vi "Spectral Integration Fast Version.vi"() -> ()   [LabVIEW 2018]
uses:
  <vilib>/Utility/file.llb/Write To Spreadsheet File (string).vi
  <vilib>/Utility/file.llb/Write To Spreadsheet File (DBL).vi
  <instrlib>/Ocean Optics 2000 4000/Ocean Optics 2000 4000.lvlib
panel:
  in  "?":bool
  out "Calculated Dlambda":dbl[][](array[numeric])
  in  "Number of Measurements":dbl=50.0
  out "Spectrum Data":dbl[][](array[numeric])
  in  "File Name":string="Example.xls" caption="add .xls for excel or .tdms, etc"
  in  "Enable Spectrum Log":bool caption="Log Data"
  out "x dlambda":dbl[](array[numeric])
  out "Spectrum":dbl[](array[numeric])
  in  "dlambda, pm, default 271pm":dbl=271.0
  out "Spectrum by Pixel Number":dbl[](array[numeric])
  out "Wavelength (nm)":dbl[](array[numeric])
  out "Spectral Integration":dbl
  in  "Integration Time, ms":dbl=100.0
  in  "Enable Strobe (Disabled)":bool
  out "Spectral Waveform":cluster{dbl[], dbl[]}(graph)
  in  "VISA resource name":refnum<visa-resource-name>
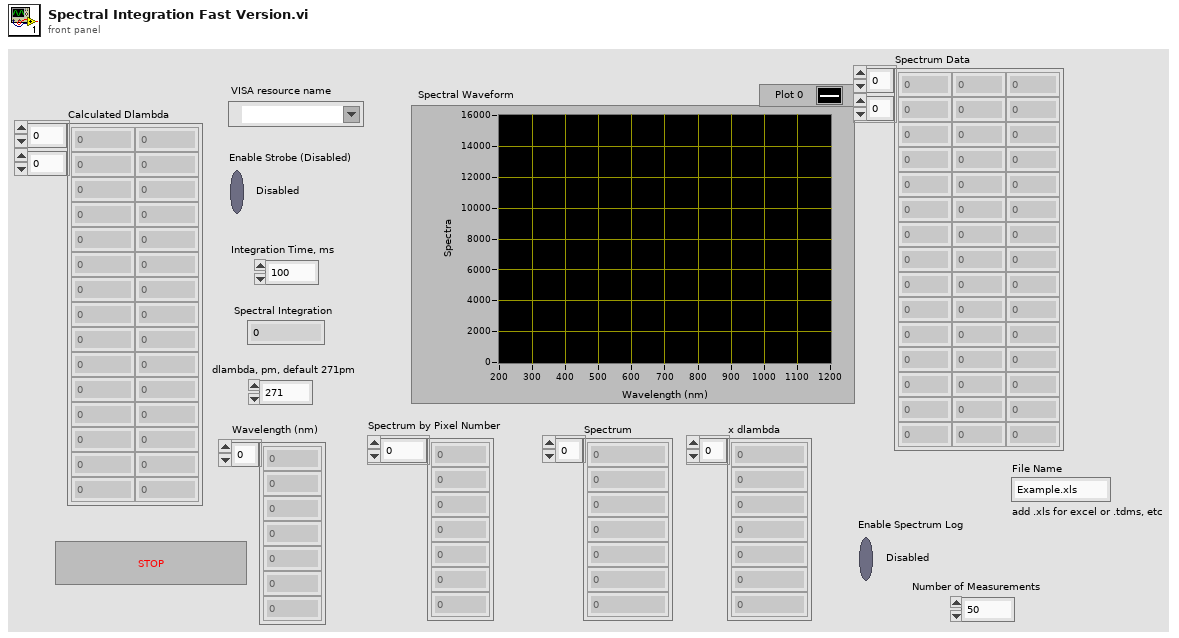
[diagram p1: front panel]
types:
  T1 = cluster{"Wavelength (nm)":dbl[], "Spectrum by Pixel Number":dbl[]}
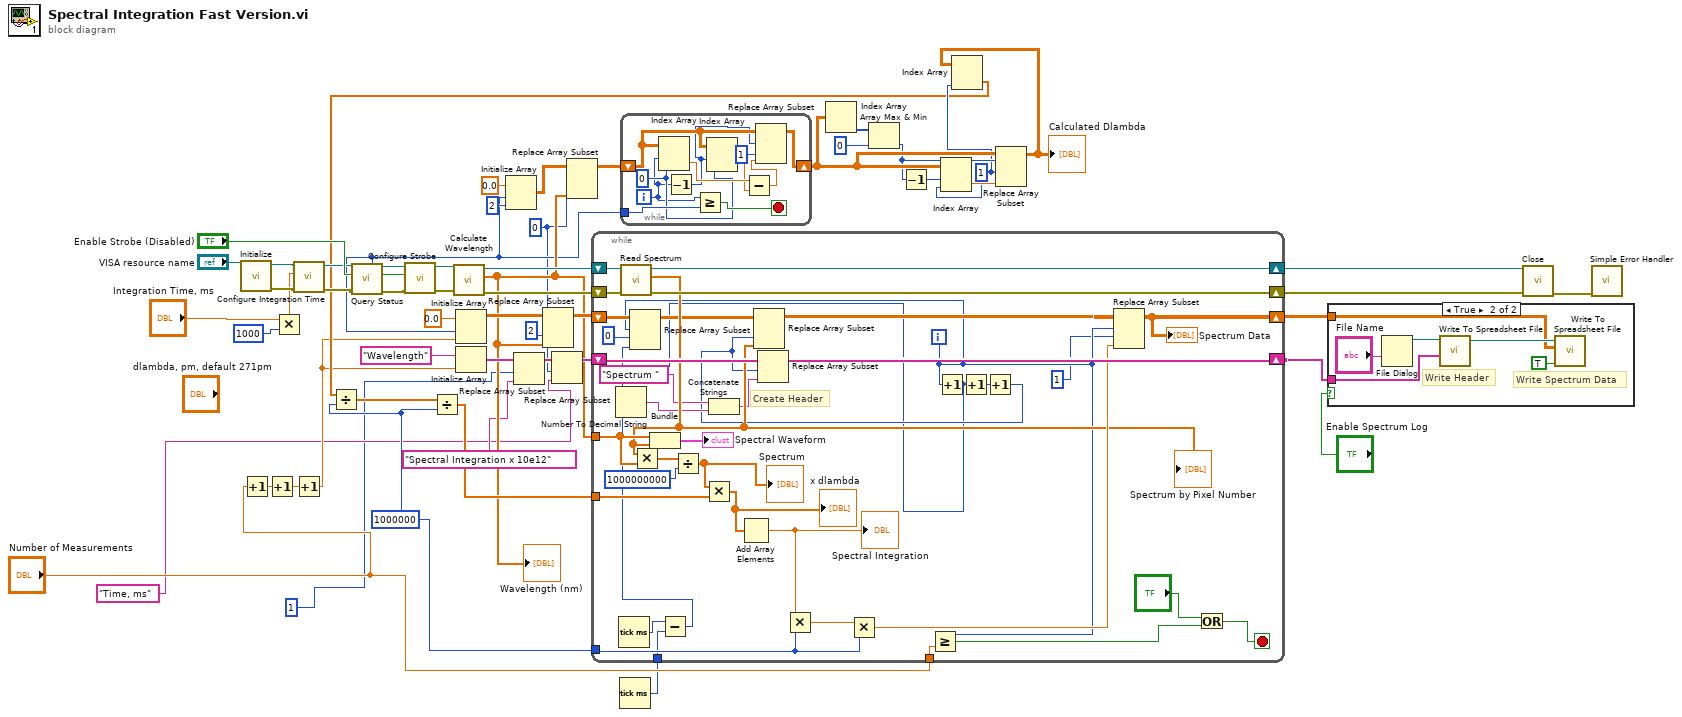
[diagram p0: block diagram]
diagram:
  w16 = 1
  w3 = 0
  w28 = 1000000
  n1 = call <instrlib>:"Initialize.vi"("VISA resource name"="VISA resource name") -> ("error out"=w51:errorcluster, "VISA resource name out"=w52:refnum<visa-resource-name>)  [unwired: 2 in, 7 out]
  n2 = Increment(x="Number of Measurements") -> (x+1=w1:dbl)
  n3 = Increment(x=w1) -> (x+1=w10:dbl)
  n4 = Multiply(x="Integration Time, ms", y=1000) -> (x*y=w48:dbl)
  n5 = call <instrlib>:"Configure Integration Time.vi"("error in (no error)"=w51, "Integration Time (6000)"=w48, "VISA resource name"=w52) -> ("error out"=w46:errorcluster, "VISA resource name out"=w44:refnum<visa-resource-name>)  [unwired: 7 in]
  n6 = Increment(x=w10) -> (x+1=w11:dbl)
  n7 = call <instrlib>:"Query Status.vi"("VISA resource name"=w44, "error in (no error)"=w46) -> ("Number of Pixels"=w14:u16, "VISA resource name out"=w43:refnum<visa-resource-name>, "error out"=w45:errorcluster)  [unwired: 11 out]
  n8 = call <instrlib>:"Configure Strobe.vi"("error in (no error)"=w45, "Enable Strobe (Disabled)"="Enable Strobe (Disabled)", "VISA resource name"=w43) -> ("error out"=w53:errorcluster, "VISA resource name out"=w54:refnum<visa-resource-name>)  [unwired: 7 out]
  n9 = call <instrlib>:"Calculate Wavelength.vi"("error in (no error)"=w53, "VISA resource name"=w54) -> ("error out"=w41:errorcluster, "Wavelength (nm)"=w15:dbl[], "VISA resource name out"=w42:refnum<visa-resource-name>)  [unwired: 1 in, 6 out]
  "Wavelength (nm)" <- w15
  n10 = Initialize Array(0.0 ("element"), w14, w11) -> (w36:dbl[][])
  n11 = Initialize Array("Wavelength", w11) -> (w30:string[])
  n12 = Initialize Array(0.0 ("element"), w14, 2) -> (w25:dbl[][])
  n13 = Replace Array Subset(array=w36, new element=w15, index (col)=2) -> (w35:dbl[][])  [unwired: 1 in]
  n14 = Replace Array Subset(array=w25, new element=w15, index (col)=w3) -> (w24:dbl[][])  [unwired: 1 in]
  n15 = Tick Count (ms)() -> (millisecond timer value=w9:u32)
  n16 = while {
    tunnel: w14 -> [w67]
    shift-right: [w61] -> w20
    shift-left: w24 -> [w63]
    i -> [w57]
    stop <- w66 stop-if-true
    w62 = 0
    n17 = Index Array(array=w63, index (row)=w57, index (col)=w62) -> (element=w65:dbl)
    n18 = Decrement(x=w57) -> (x-1=w58:i32)
    n19 = Greater Or Equal?(x=w57, y=w67) -> (x >= y?=w66:bool)
    n20 = Index Array(array=w63, index (row)=w58, index (col)=w62) -> (element=w64:dbl)
    n21 = Subtract(x=w65, y=w64) -> (x-y=w59:dbl)
    n22 = Replace Array Subset(array=w63, new element=w59, index (row)=w58, index (col)=1) -> (w61:dbl[][])
  }
  n23 = Array Max & Min(array=w20) -> (min index (indices)=w23:i32[])  [unwired: 3 out]
  n24 = Index Array(array=w23, index=0) -> (element=w18:i32)
  n25 = Decrement(x=w18) -> (x-1=w22:i32)
  n26 = Index Array(array=w20, index (row)=w22, index (col)=w16) -> (element=w21:dbl)
  n27 = Replace Array Subset(array=w20, new element=w21, index (row)=w18, index (col)=w16) -> (w19:dbl[][])
  "Calculated Dlambda" <- w19
  n28 = Index Array(array=w19, index (col)=w16) -> (element=w13:dbl[])  [unwired: 1 in]
  n29 = Divide(x=w13, y=w28) -> (x/y=w37:dbl[])
  n30 = Divide(x=w37, y=w28) -> (x/y=w34:dbl[])
  n31 = while {
    tunnel: w15 -> [w98]
    tunnel: w34 -> [w103]
    tunnel: w28 -> [w94]
    shift-right: [w86] -> w40
    shift-left: w42 -> [w90]
    shift-right: [w88] -> w39
    shift-left: w41 -> [w91]
    shift-right: [w97] -> w29
    shift-left: w35 -> [w92]
    tunnel: "Number of Measurements" -> [w80]
    tunnel: w9 -> [w78]
    shift-right: [w73] -> w8
    shift-left: w30 -> [w93]
    i -> [w74]
    stop <- w68 stop-if-true
    # "Create Header"
    n32 = Tick Count (ms)() -> (millisecond timer value=w81:u32)
    n33 = call <instrlib>:"Read Spectrum.vi"("error in (no error)"=w91, "VISA resource name"=w90) -> ("error out"=w88:errorcluster, "Spectrum by Pixel Number"=w87:dbl[], "VISA resource name out"=w86:refnum<visa-resource-name>)  [unwired: 6 in, 1 out]
    "Spectrum by Pixel Number" <- w87
    n34 = Multiply(x=w87, y=w98) -> (x*y=w101:dbl[])
    n35 = Bundle("Wavelength (nm)"=w98, "Spectrum by Pixel Number"=w87) -> (→"Spectral Waveform":T1)  [unwired: 1 out]
    n36 = Subtract(x=w81, y=w78) -> (x-y=w76:u32)
    n37 = Replace Array Subset(array=w92, new element=w76, index (row)=w74, index (col)=0) -> (w77:dbl[][])
    n38 = Divide(x=w101, y=1000000000) -> (x/y=w99:dbl[])
    "Spectrum" <- w99
    n39 = Multiply(x=w99, y=w103) -> (x*y=w104:dbl[])
    "x dlambda" <- w104
    n40 = Add Array Elements(numeric array=w104) -> (sum=w102:dbl)
    "Spectral Integration" <- w102
    n41 = Multiply(x=w102, y=w94) -> (x*y=w96:dbl)
    n42 = Multiply(x=w96, y=w94) -> (x*y=w95:dbl)
    n43 = Greater Or Equal?(x=w74, y=w80) -> (x >= y?=w70:bool)
    n44 = Increment(x=w74) -> (x+1=w71:i32)
    n45 = Number To Decimal String(number=w71) -> (decimal integer string=w85:string)  [unwired: 1 out]
    n46 = Concatenate Strings("Spectrum " ("string"), w85) -> (w83:string)
    n47 = Increment(x=w71) -> (x+1=w79:i32)
    n48 = Increment(x=w79) -> (x+1=w82:i32)
    n49 = Replace Array Subset(array=w77, new element=w87, index (col)=w82) -> (w89:dbl[][])  [unwired: 1 in]
    n50 = Replace Array Subset(array=w93, new element=w83, index=w82) -> (w73:string[])
    n51 = Replace Array Subset(array=w89, new element=w95, index (row)=w74, index (col)=1) -> (w97:dbl[][])
    "Spectrum Data" <- w97
    n52 = Or(x="?", y=w70) -> (x .or. y?=w68:bool)
  }
  n53 = Replace Array Subset(array=w8, new element="Spectral Integration x 10e12" ("string"), index=1) -> (w7:string[])
  n54 = Replace Array Subset(array=w7, new element="Time, ms" ("string"), index=w3) -> (w5:string[])
  n55 = case shown="True" "Enable Spectrum Log" {
    tunnel: w29 -> [_ w108]
    tunnel: w5 -> [_ w106]
    frame False {
    }
    frame True {
      # "Write Spectrum Data"
      # "Write Header"
      n56 = File Dialog(9:"File Name") -> (3:w110:path)  [unwired: 1 in, 8 out]
      n57 = call-poly <vilib>:"Write To Spreadsheet File.vi"("1D data"=w106, "file path (dialog if empty)"=w110) -> ("new file path (Not A Path if cancelled)"=w109:path)  [unwired: 4 in, 2 out]
      n58 = call-poly <vilib>:"Write To Spreadsheet File.vi"("append to file? (new file:F)"=TRUE, "2D data"=w108, "file path (dialog if empty)"=w109) -> ()  [unwired: 3 in, 3 out]
    }
  }
  n59 = call <instrlib>:"Close.vi"("error in (no error)"=w39, "VISA resource name"=w40) -> ("error out"=w38:errorcluster)  [unwired: 9 out]
  n60 = call <vilib>:"Simple Error Handler.vi"("error in (no error)"=w38) -> ()  [unwired: 2 in, 7 out]
